vi "Test Client to Server (TCP).vi"(0 "port":u16, 2 "Stop":bool, 3 "error in (no error)":errorcluster) -> (7 "Results":T1, 8 "Test Finished?":bool, 10 "error out":errorcluster)   [LabVIEW 2019]
doc: "Tests ports in direction of cliend to server"
uses:
  controls/Results.ctl
  controls/Log Data Cluster.ctl
  controls/Communication Types.ctl
panel:
  in  "Message to Send":string="You are currently accessing TCP Named Service - Server.vi from client %s on port %d."
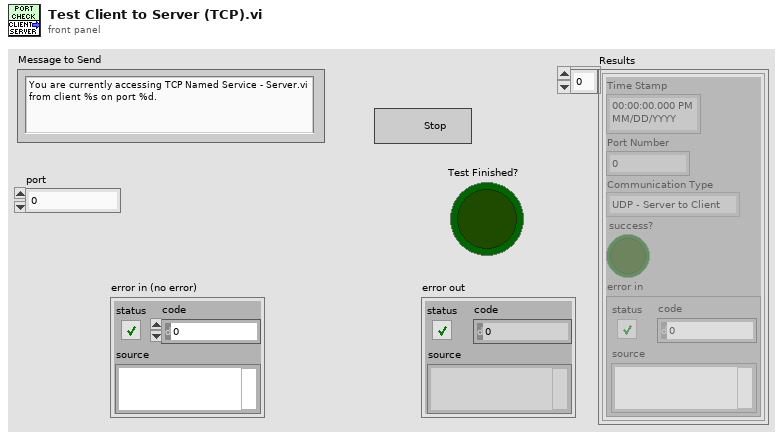
[diagram p1: front panel]
types:
  T1 = typedef "Results.ctl" = T2[]
  T2 = typedef "log data cluster.ctl" = cluster{"Time Stamp":timestamp, "Port Number":u16, "Communication Type":T3, "success?":bool, "error in":errorcluster}
  T3 = typedef "Communication Types.ctl" = enum16{"UDP - Server to Client", "UDP - Client to Server", "TCP - Server to Client", "TCP - Client to Server"}
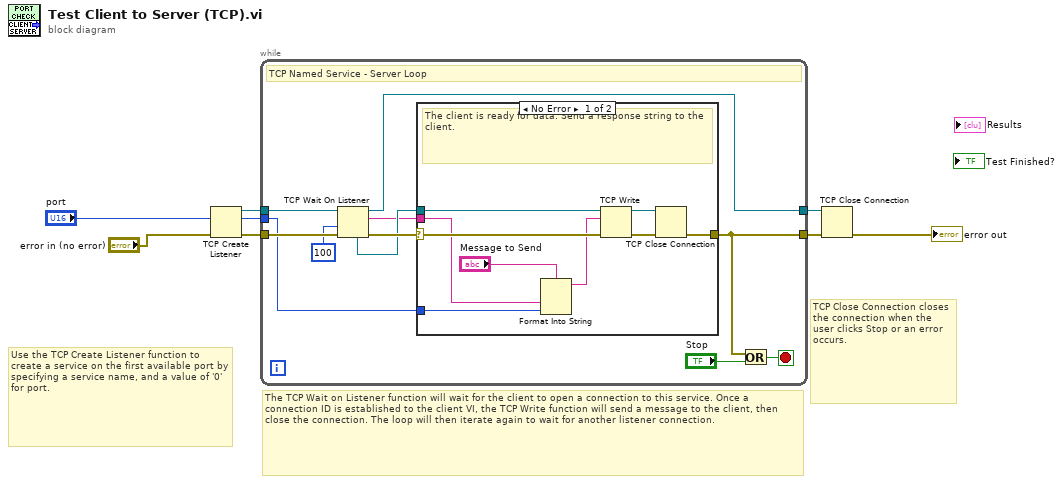
[diagram p0: block diagram]
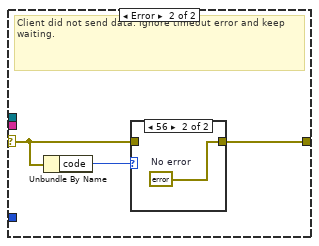
[diagram p2: hidden frame]
diagram:
  # "TCP Close Connection closes the connection when the user clicks Stop or an error occurs."
  # "The TCP Wait on Listener function will wait for the client to open a connection to this service. Once a connection ID is established to the client VI, the TCP Write function will send a message to the client, then close the connection. The loop will then iterate again to wait for another listener connection."
  # "Use the TCP Create Listener function to create a service on the first available port by specifying a service name, and a value of '0' for port."
  n1 = TCP Create Listener(8:"error in (no error)", 10:"port") -> (0:w7:errorcluster, 2:w4:u16, 3:w8:refnum<k5>)  [unwired: 3 in]
  n2 = while {
    tunnel: [w12] -> w5
    tunnel: w8 -> [w19]
    tunnel: w7 -> [w17]
    tunnel: [w9] -> w6
    tunnel: w4 -> [w15]
    stop <- w14 stop-if-true
    # "TCP Named Service - Server Loop"
    n3 = TCP Wait On Listener(8:w17, 9:100 ("timeout ms (25000)"), 11:w19) -> (0:w18:errorcluster, 2:w10:string, 3:w9:refnum<k5>, 4:w16:refnum<k5>)  [unwired: 1 in, 1 out]
    n4 = case shown="No Error" w18 {
      selector: w18 -> [w28 w31]
      tunnel: [w21 w29] -> w12
      tunnel: w16 -> [w22 _]
      tunnel: w15 -> [w26 _]
      tunnel: w10 -> [w24 _]
      frame No Error {
        # "The client is ready for data. Send a response string to the client."
        n5 = Format Into String(format string="Message to Send", w24, w26) -> (resulting string=w23:string)  [unwired: 2 in, 1 out]
        n6 = TCP Write(connection ID=w22, data in=w23, error in (no error)=w28) -> (connection ID out=w20:refnum<k5>, error out=w27:errorcluster)  [unwired: 1 in, 1 out]
        n7 = TCP Close Connection(connection ID=w20, error in (no error)=w27) -> (error out=w21:errorcluster)  [unwired: 1 in, 1 out]
      }
      frame Error {
        # "Client did not send data. Ignore timeout error and keep waiting."
        n8 = Unbundle By Name(w31) -> ("code"=w30:i32)
        n9 = case shown="56" w30 {
          tunnel: w31 -> [w32 _]
          tunnel: [w32 w33] -> w29
          frame Default {
          }
          frame 56 {
            w33 = errorcluster {"status"=FALSE, "code"=0, "source"=""}  # No error
          }
        }
      }
    }
    n10 = Or(x=w12, y="Stop") -> (x .or. y?=w14:bool)
  }
  n11 = TCP Close Connection(connection ID=w6, error in (no error)=w5) -> (error out=→"error out":errorcluster)  [unwired: 1 in, 1 out]
